vi "Create Advanced Sequence Name.vi"(0 "Channel Name":string, 11 "error in (no error)":errorcluster) -> (4 "String":string, 15 "error out":errorcluster)   [LabVIEW 2024, in "devicePowerSequencerCoreLogic.lvlib"]
uses:
  devicePowerSequencerCoreLogic.lvlib
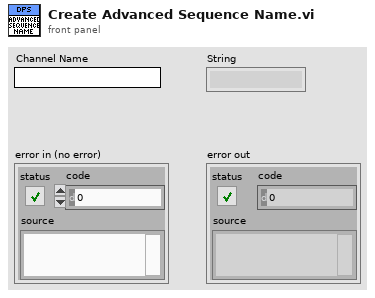
[diagram p1: front panel]
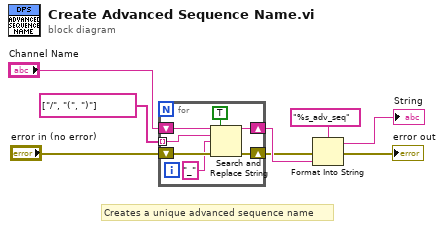
[diagram p0: block diagram]
diagram:
  # "Creates a unique advanced sequence name"
  n1 = for {
    shift-right: [w14] -> w5
    shift-left: "error in (no error)" -> [w15]
    shift-right: [w11] -> w7
    shift-left: "Channel Name" -> [w10]
    tunnel: string[] ["/", "(", ")"] -> [w9] mode=indexing
    n2 = Search and Replace String(replace all?=TRUE ("replace all? (F)"), input string=w10, search string=w9, replace string="_" ("replace string (\"\")"), error in=w15) -> (result string=w11:string, error out=w14:errorcluster)  [unwired: 3 in, 2 out]
  }
  n3 = Format Into String(format string="%s_adv_seq", error in=w5, w7) -> (resulting string=→"String":string, error out=→"error out":errorcluster)  [unwired: 1 in]
